vi "Find String with Option.vi"(8 "error in (no error)":errorcluster caption="错误输入（无错误）", 9 "options":i32(ring) items=["None"=0, "WholeWord"=2, "MatchCase"=4, "NoHighlight"=8, "Reverse"=16], 10 "str":string, 11 "RichText 输入":refnum<class "RichText.lvclass"> caption="DNL_LabVIEW Object in") -> (0 "error out":errorcluster caption="错误输出", 2 "Find":i32, 3 "RichText 输出":refnum<class "RichText.lvclass"> caption="DNL_LabVIEW Object out")   [LabVIEW 2012, in "RichText.lvclass"]
uses:
  RichText.lvclass
  RichText.lvclass/RichText.ctl
  System.Windows.Forms
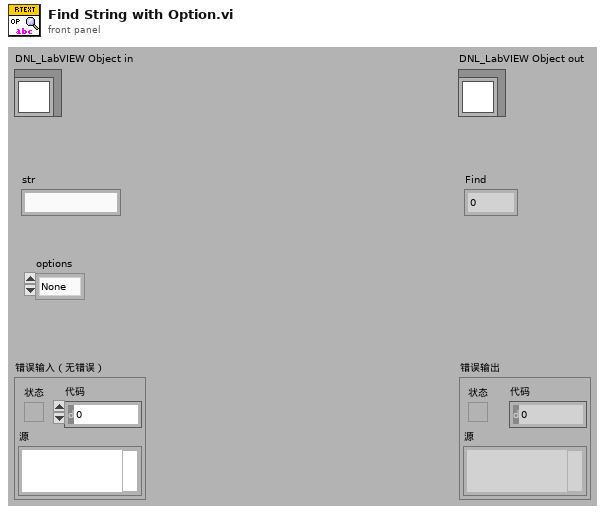
[diagram p1: front panel]
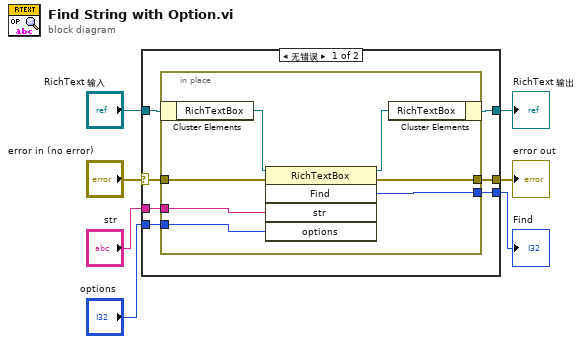
[diagram p0: block diagram]
diagram:
  n1 = case shown="无错误" "error in (no error)" {
    selector: "error in (no error)" -> [w10 w23]
    tunnel: [w9 w23] -> w6
    tunnel: [w11 w22] -> w4
    tunnel: "RichText 输入" -> [w14 w22]
    tunnel: "str" -> [w13 _]
    tunnel: "options" -> [w12 _]
    tunnel: [w8 _] -> w1
    frame No Error {
      n2 = in-place {
        in-place-border: w13 -> [w19]
        in-place-border: w12 -> [w18]
        in-place-border: w10 -> [w17]
        in-place-border: [w16] -> w9
        in-place-border: [w15] -> w8
        n3 = in-place-cluster #1(w14) -> ("RichTextBox"=w21:refnum<k24>)
        n4 = invoke class="RichTextBox" method="Find"(reference=w21, error in=w17, "str"=w19, "options"=w18) -> (reference out=w20:refnum<k24>, error out=w16:errorcluster, "Find"=w15:i32)  [unwired: 1 in, 2 out]
        n5 = in-place-cluster #1("RichTextBox"=w20) -> (w11:refnum<class "RichText.lvclass">)
      }
    }
    frame Error {
    }
  }
  "error out" <- w6
  "RichText 输出" <- w4
  "Find" <- w1
